vi "gd_branches_builder.vi"(7 "GD":bool, 10 "Event type":string="GL") -> (3 "GD branches":string)   [LabVIEW 2020]
uses:
  <vilib>/Utility/file.llb/Read Delimited Spreadsheet (string).vi
panel:
  out "GDs nodes":string[](array[string])
  in  "Lista de condições (arquivo.txt) 2":string="list_GDs.txt"
  in  "Diretório de trabalho":path=path "C:/ATP/ATPDraw/Projects_Flavio"
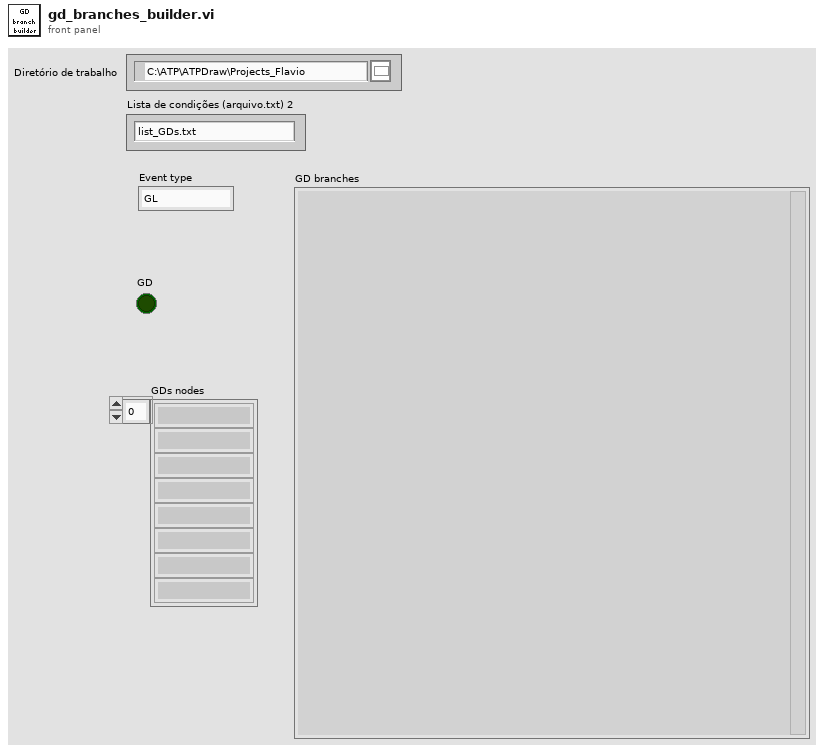
[diagram p1: front panel]
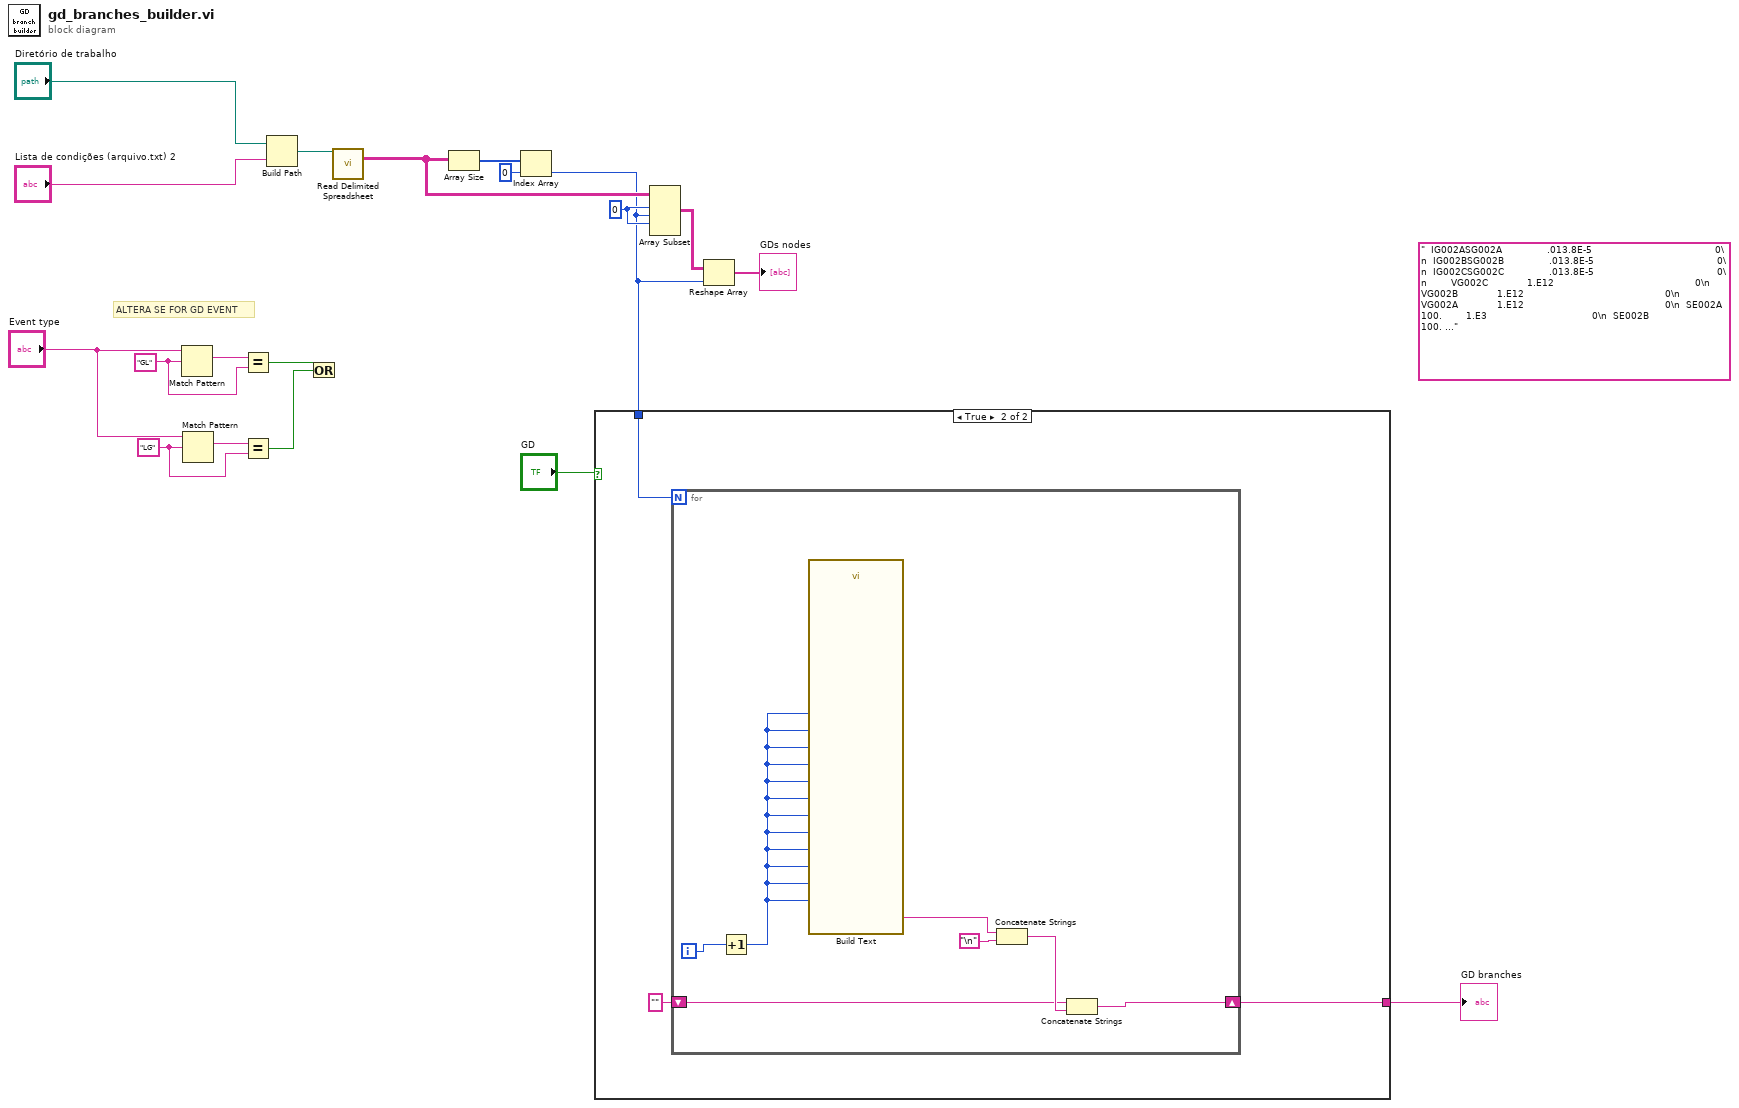
[diagram p0: block diagram]
diagram:
  w9 = 0 ("index")
  (unwired) "  IG002ASG002A               .013.8E-5                                         0\n  IG002BSG002B               .013.8E-5                                         0\n  IG002CSG002C               .013.8E-5                                         0\n        VG002C             1.E12                                               0\n        VG002B             1.E12                                               0\n        VG002A             1.E12                                               0\n  SE002A                    100.        1.E3                                   0\n  SE002B                    100.        1.E3                                   0\n  SE002C                    100.        1.E3                                   0"
  w18 = "GL" ("regular expression")
  w16 = "LG" ("regular expression")
  # "ALTERA SE FOR GD EVENT"
  n1 = Match Pattern(string="Event type", regular expression=w18) -> (match substring=w17:string)  [unwired: 1 in, 3 out]
  n2 = Match Pattern(string="Event type", regular expression=w16) -> (match substring=w19:string)  [unwired: 1 in, 3 out]
  n3 = Equal?(x=w17, y=w18) -> (x = y?=w14:bool)
  n4 = Equal?(x=w19, y=w16) -> (x = y?=w15:bool)
  n5 = Build Path(base path="Diretório de trabalho", name or relative path="Lista de condições (arquivo.txt) 2") -> (appended path=w11:path)
  n6 = Or(x=w14, y=w15) -> ()  [unwired: 1 out]
  n7 = call-poly <vilib>:"Read Delimited Spreadsheet.vi"("file path (dialog if empty)"=w11) -> ("all rows"=w8:string[][])  [unwired: 9 in, 5 out]
  n8 = Array Size(array=w8) -> (size(s)=w7:i32[])
  n9 = Index Array(array=w7, index=0) -> (element=w2:i32)
  n10 = case shown="True" "GD" {
    tunnel: [_ w22] -> w12
    tunnel: w2 -> [_ w21]
    frame False {
    }
    frame True {
      n11 = for {
        N: w21 -> [_]
        shift-right: [w23] -> w22
        shift-left: "" -> [w24]
        i -> [w29]
        n12 = Increment(x=w29) -> (x+1=w28:i32)
        n13 = call "Build Text"("ig_a"=w28, "sg_a"=w28, "ig_b"=w28, "sg_b"=w28, "ig_c"=w28, "sg_c"=w28, "vg_a"=w28, "vg_b"=w28, "vg_c"=w28, "se_a"=w28, "se_b"=w28, "se_c"=w28) -> ("Result"=w25:string)  [unwired: 14 in, 1 out]
        n14 = Concatenate Strings(w25, "\n") -> (w26:string)
        n15 = Concatenate Strings(w24, w26) -> (w23:string)
      }
    }
  }
  "GD branches" <- w12
  n16 = Array Subset(array=w8, index (row)=w9, length (row)=w2, index (col)=w9) -> (w5:string[][])  [unwired: 1 in]
  n17 = Reshape Array(w5, w2) -> (→"GDs nodes":string[])
